vi "OpenG Array filter - Regexp Invert Array Template.vi"() -> ()   [LabVIEW 2018]
panel:
  out "filtered item indices":i32[](array[numeric])
  out "filtered array":string[](array[string])
  in  "items to filter":string[](array[string])
  in  "Array Input":string[](array[string])
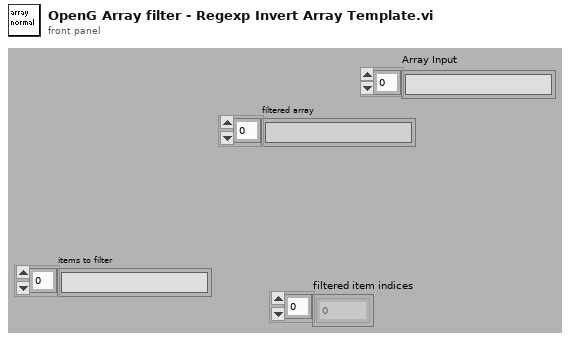
[diagram p1: front panel]
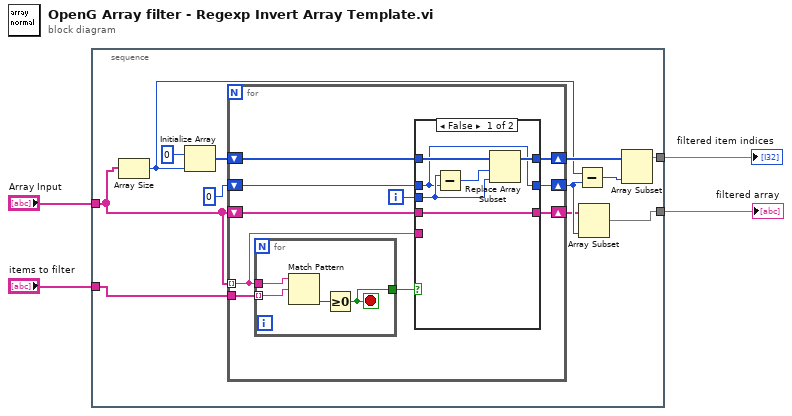
[diagram p0: block diagram]
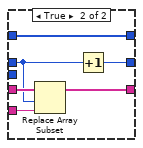
[diagram p2: hidden frame]
diagram:
  n1 = stacked-sequence {
    tunnel: "items to filter" -> [w7]
    tunnel: [w6] -> w3
    tunnel: "Array Input" -> [w8]
    tunnel: [w5] -> w1
    frame #0 {
      n2 = Array Size(array=w8) -> (size(s)=w13:i32)
      n3 = Initialize Array(0 ("Numeric"), w13) -> (w12:i32[])
      n4 = for {
        tunnel: w8 -> [w23] mode=indexing
        shift-right: [w24] -> w10
        shift-left: w8 -> [w26]
        shift-right: [w21] -> w15
        shift-left: 0 -> [w22]
        shift-right: [w19] -> w14
        shift-left: w12 -> [w20]
        tunnel: w7 -> [w18]
        i -> [w17]
        n5 = for {
          tunnel: [w29] -> w25
          tunnel: w23 -> [w28]
          tunnel: w18 -> [w27] mode=indexing
          stop <- w29 stop-if-true
          n6 = Match Pattern(string=w28, regular expression=w27) -> (offset past match=w30:i32)  [unwired: 4 out]
          n7 = Greater Or Equal To 0?(x=w30) -> (x >= 0?=w29:bool)
        }
        n8 = case shown="False" w25 {
          tunnel: w26 -> [w36 w42]
          tunnel: [w36 w41] -> w24
          tunnel: w23 -> [_ w40]
          tunnel: w22 -> [w32 w38]
          tunnel: [w32 w39] -> w21
          tunnel: w20 -> [w35 w37]
          tunnel: [w34 w37] -> w19
          tunnel: w17 -> [w33 _]
          frame False {
            n9 = Subtract(x=w33, y=w32) -> (x-y=w31:i32)
            n10 = Replace Array Subset(array=w35, new element=w33, index=w31) -> (w34:i32[])
          }
          frame True {
            n11 = Replace Array Subset(array=w42, new element=w40, index=w38) -> (w41:string[])
            n12 = Increment(x=w38) -> (x+1=w39:i32)
          }
        }
      }
      n13 = Subtract(x=w13, y=w15) -> (x-y=w16:i32)
      n14 = Array Subset(array=w10, length=w15) -> (w5:string[])  [unwired: 1 in]
      n15 = Array Subset(array=w14, length=w16) -> (w6:i32[])  [unwired: 1 in]
    }
  }
  "filtered array" <- w1
  "filtered item indices" <- w3
